vi "TestRFGVAck.vi"() -> (0 "error out":errorcluster, 2 "Pass":bool)   [LabVIEW 2015]
uses:
  TypeDef/RequestActionEnum.ctl
  LVClasses/Request/PersonnelType.ctl
  TypeDef/PersonnelAndTime.ctl
  TypeDef/Limits.ctl
  LVClasses/Request/Request.lvclass/Request.ctl
  LVClasses/Request/Read AckName.vi
  LVClasses/Request/Read AckTime.vi
  LVClasses/Request/Request.lvclass
panel:
  out "TimeStamp":bool
  out "Name":bool
  out "Request":string
  out "Add Request":string
  out "Ack":string
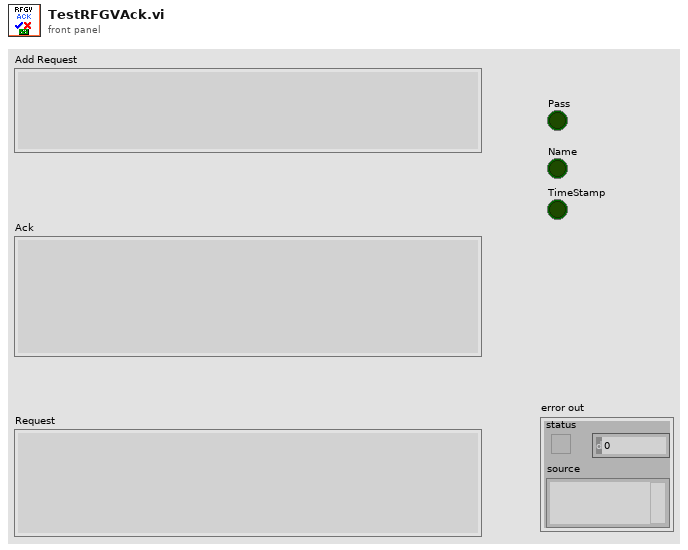
[diagram p1: front panel]
types:
  T1 = typedef "Limits.ctl" = cluster{"AckLimit":dbl, "CompleteLimit":dbl}
  T2 = typedef "PersonnelAndTime.ctl" = cluster{"Personnel":string, "TimeStamp":string}
  T3 = typedef "RequestActionEnum.ctl" = enum16{"Init", "ReadRequests", "ReadRequest", "AddRequest", "RemoveRequest", "ToDisk", "Ack", "Complete", "CheckAlarms", "PIntoRoom", "Read Summary", "GetRequestForRoom"}
  T4 = typedef "Request.lvclass/PersonnelType.ctl" = u16
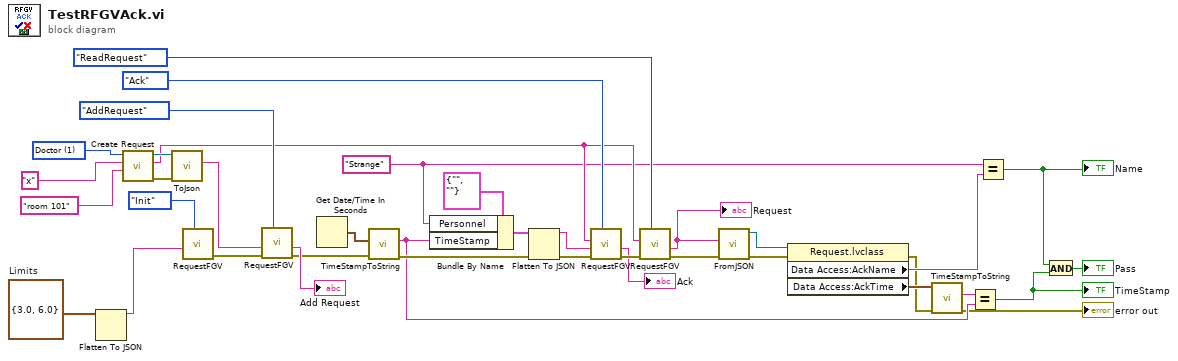
[diagram p0: block diagram]
diagram:
  w2 = T1 {"AckLimit"=3.0, "CompleteLimit"=6.0}  # Limits
  w9 = "Strange" ("Personnel")
  w31 = T4 1 items=["Nurse", "Doctor", "Cleanning", "Admin"] ("Type 2")
  n1 = Flatten To JSON(anything=w2) -> (JSON string=w1:string)  [unwired: 2 in, 1 out]
  n2 = call "Create Request.vi"("Description"="room 101" (".Description 2"), "Name"="x" ("Name 2"), "Personnel Type"=w31) -> ("error out"=w36:errorcluster, "RUID"=w16:string, "Request out"=w35:refnum<class "Request.lvclass">)  [unwired: 6 in]
  n3 = call "ToJson.vi"("error in (no error)"=w36, "Request"=w35) -> ("Request"=w34:string)  [unwired: 8 in, 1 out]
  n4 = call "RequestFGV.vi"("Actions"=RequestActionEnum."Init", "Data In"=w1) -> ("error out"=w28:errorcluster)  [unwired: 8 in, 1 out]
  n5 = call "RequestFGV.vi"("Actions"=RequestActionEnum."AddRequest", "error in (no error)"=w28, "Data In"=w34) -> ("error out"=w18:errorcluster, "Data Out"=→"Add Request":string)  [unwired: 7 in]
  n6 = Get Date/Time In Seconds() -> (seconds since 1Jan1904=w24:timestamp)
  n7 = call "TimeStampToString.vi"("error in (no error)"=w18, "Time Stamp"=w24) -> ("error out"=w20:errorcluster, "String"=w11:string)  [unwired: 8 in]
  n8 = Bundle By Name(cluster=T2 {"Personnel"="", "TimeStamp"=""}, "Personnel"=w9, "TimeStamp"=w11) -> (w23:T2)
  n9 = Flatten To JSON(anything=w23, error in (no error)=w20) -> (JSON string=w22:string, 11:w21:errorcluster)  [unwired: 1 in]
  n10 = call "RequestFGV.vi"("Actions"=RequestActionEnum."Ack", "error in (no error)"=w21, "Data In"=w22, "RUID"=w16) -> ("error out"=w26:errorcluster, "Data Out"=→"Ack":string)  [unwired: 6 in]
  n11 = call "RequestFGV.vi"("Actions"=RequestActionEnum."ReadRequest", "error in (no error)"=w26, "RUID"=w16) -> ("error out"=w17:errorcluster, "Data Out"=w15:string)  [unwired: 7 in]
  "Request" <- w15
  n12 = call "FromJSON.vi"("error in (no error)"=w17, "Request"=w15) -> ("error out"=w5:errorcluster, "Request out"=w14:refnum<class "Request.lvclass">)  [unwired: 8 in]
  n13 = property class="Request.lvclass"(reference=w14, error in=w5) -> (error out=w4:errorcluster, "Data Access:AckName"=w10:string, "Data Access:AckTime"=w13:timestamp)  [unwired: 1 out]
  n14 = call "TimeStampToString.vi"("error in (no error)"=w4, "Time Stamp"=w13) -> ("error out"=→"error out":errorcluster, "String"=w12:string)  [unwired: 8 in]
  n15 = Equal?(x=w12, y=w11) -> (x = y?=w7:bool)
  "TimeStamp" <- w7
  n16 = Equal?(x=w9, y=w10) -> (x = y?=w8:bool)
  "Name" <- w8
  n17 = And(x=w8, y=w7) -> (x .and. y?=→"Pass":bool)
